vi "Wire Between Unbundle And Bundle For Message Converter With Oneof.vi"(8 "error in (no error)":errorcluster, 9 "Message Metadata":T1, 10 "VI Refnum":refnum<vi>, 11 "Library ref in":refnum<vi>) -> (0 "error IO":errorcluster, 2 "VI Refnum out":refnum<vi>, 3 "Library ref out":refnum<vi>)   [LabVIEW 2019, in "gRPC Template Creation Utility.lvlib"]
uses:
  gRPC Template Creation Utility.lvlib
  TypeDefs/Message Metadata (Scripting).ctl
  TypeDefs/Message Element Metadata (Scripting).ctl
  TypeDefs/Message Element Type.ctl
  <vilib>/Utility/miscctls.llb/LVPointTypeDef.ctl
  <vilib>/Utility/Data Type/NI_Data Type.lvlib
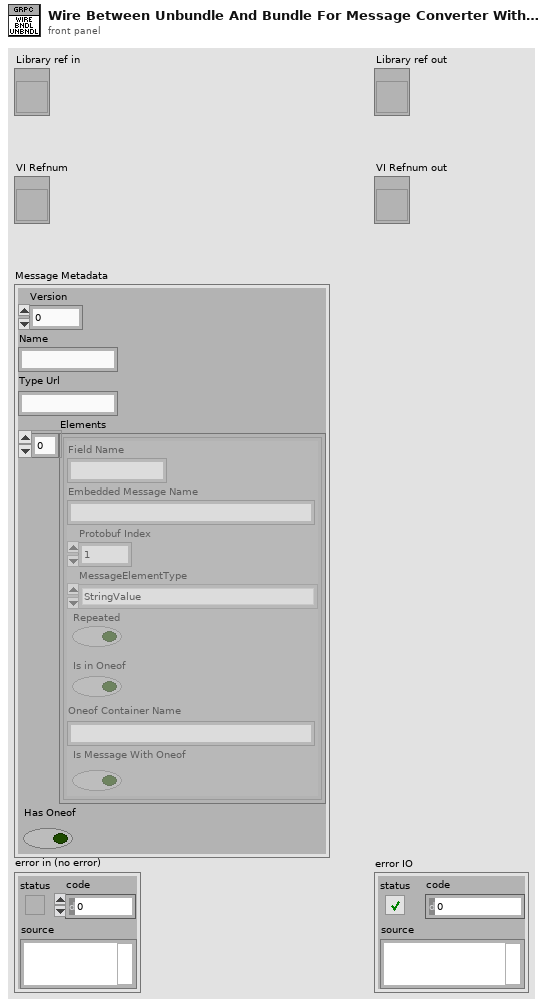
[diagram p1: front panel]
types:
  T1 = typedef "gRPC Template Creation Utility.lvlib/Message Metadata (Scripting).ctl" = cluster{"Version":i32, "Name":string, "Type Url":string, "Elements":T2[], "Has Oneof":bool}
  T2 = typedef "gRPC Template Creation Utility.lvlib/Message Element Metadata (Scripting).ctl" = cluster{"Field Name":string, "Embedded Message Name":string, "Protobuf Index":i32, "MessageElementType":T3, "Repeated":bool, "Is in Oneof":bool, "Oneof Container Name":string, "Is Message With Oneof":bool}
  T3 = typedef "gRPC Template Creation Utility.lvlib/Message Element Type.ctl" = enum32{"Int32Value", "FloatValue", "DoubleValue", "BoolValue", "StringValue", "MessageValue", "Int64Value", "UInt32Value", "UInt64Value", "EnumValue", "Bytes", "Fixed64", "Fixed32", "SFixed64", "SFixed32", "SInt64", "SInt32"}
  T4 = typedef "LVPointTypeDef.ctl" = cluster{"Horizontal":i16, "Vertical":i16}
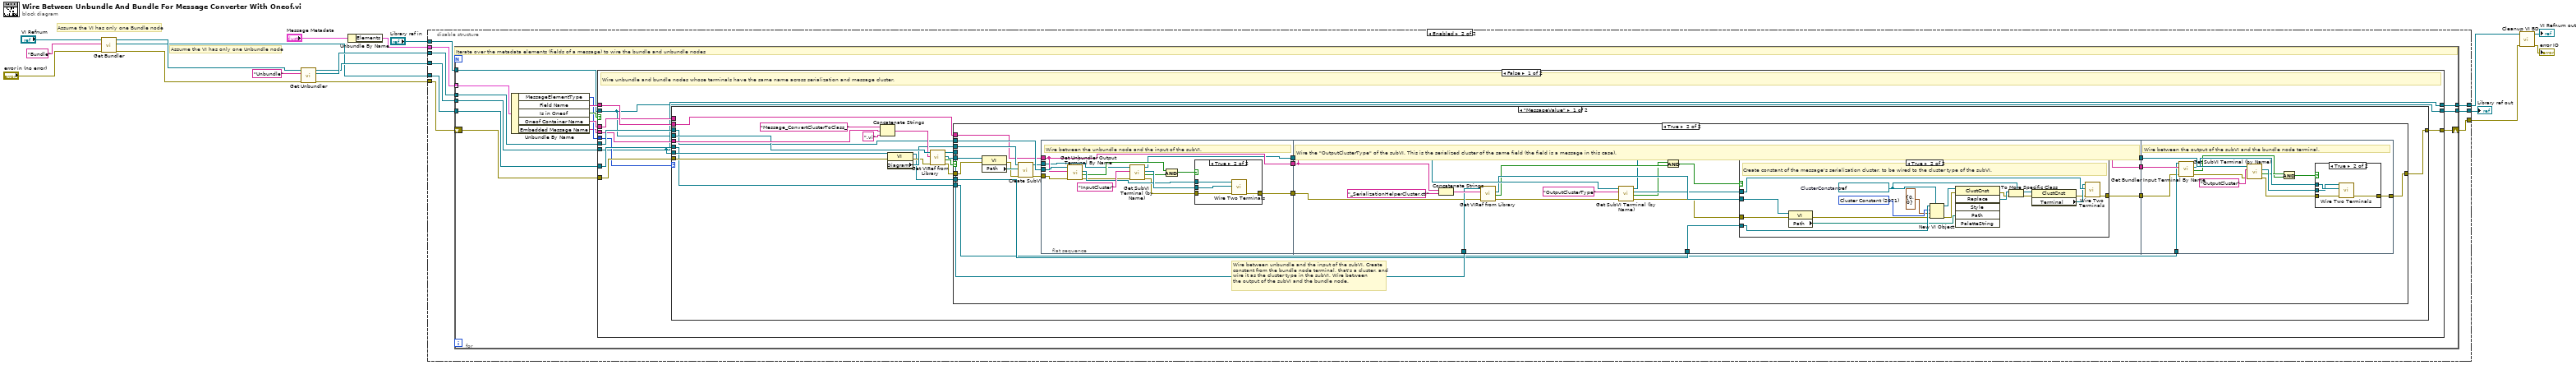
[diagram p0: block diagram]
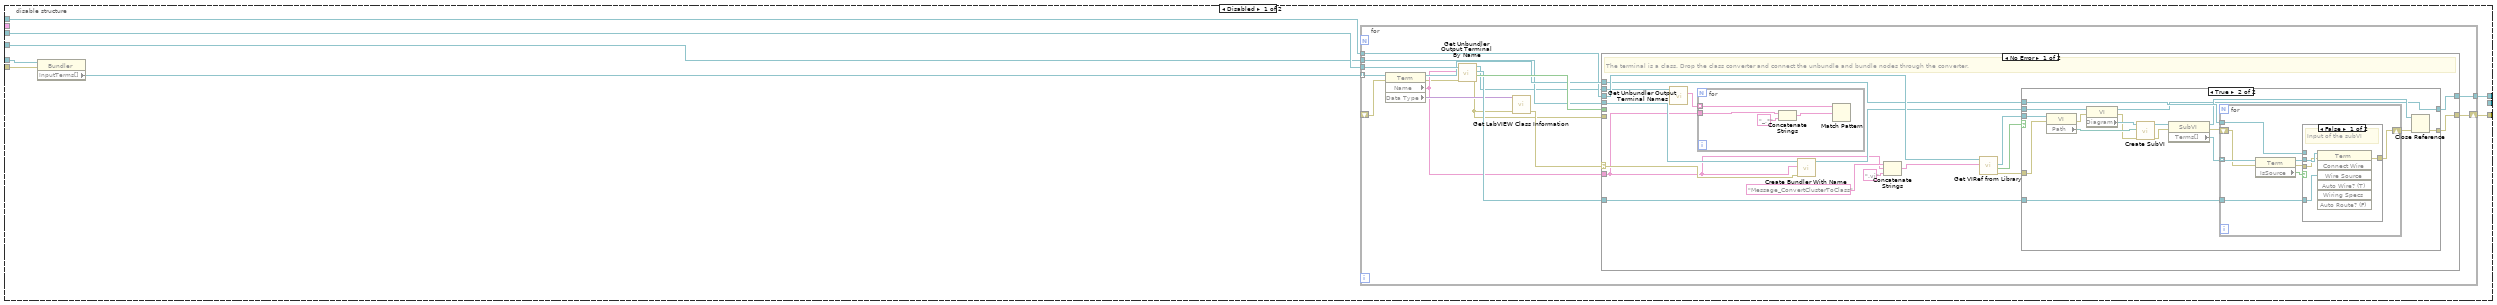
[diagram p2: hidden frame]
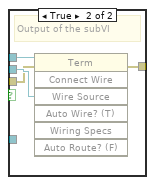
[diagram p4: hidden frame]
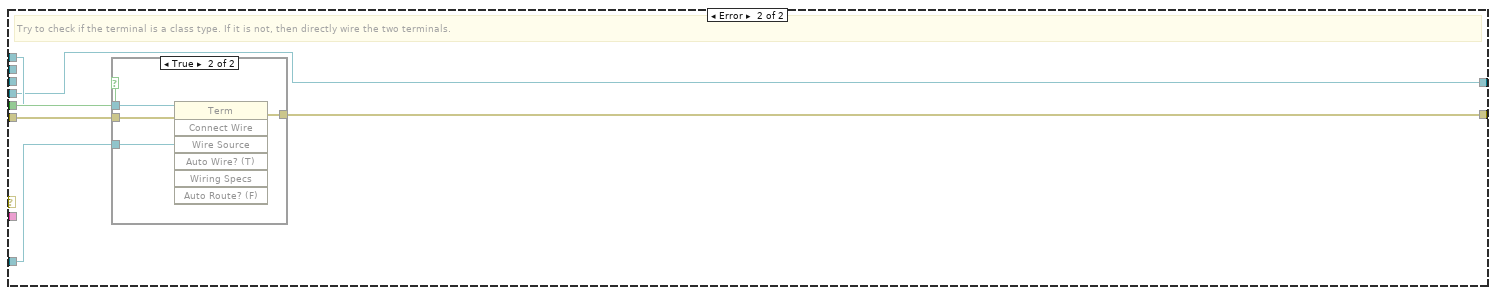
[diagram p5: hidden frame]
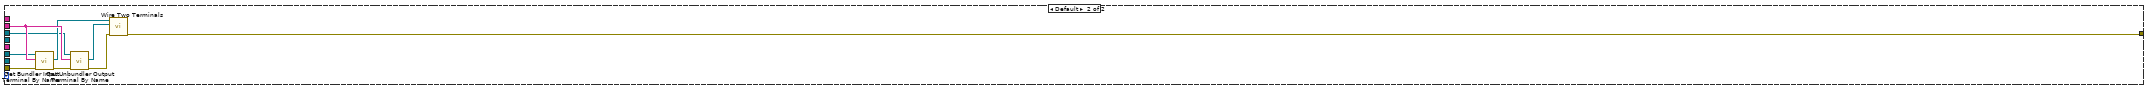
[diagram p11: hidden frame]
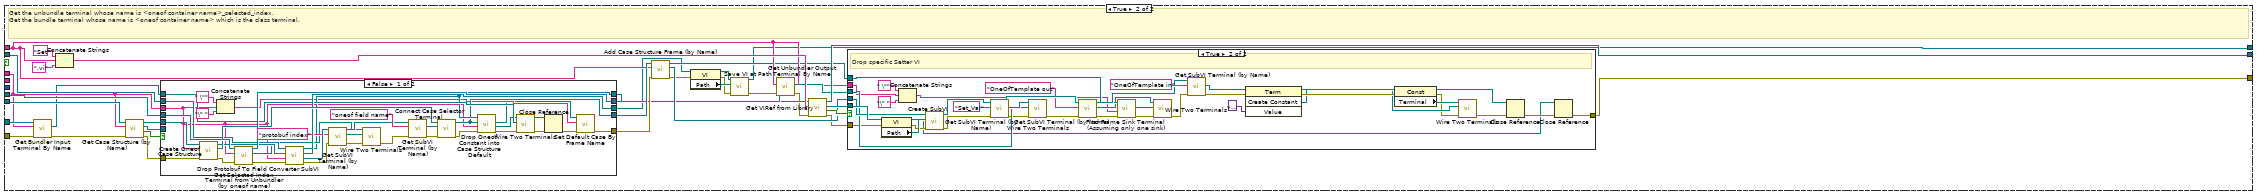
[diagram p12: hidden frame]
diagram:
  # "Assume the VI has only one Bundle node"
  # "Assume the VI has only one Unbundle node"
  n1 = call "Get Bundler.vi"("error in (no error)"="error in (no error)", "Label"="Bundle" ("Class Name"), "Owner VI in"="VI Refnum") -> ("error out"=w6:errorcluster, "Bundler ref out"=w3:refnum<vi>, "Owner VI out"=w7:refnum<vi>)  [unwired: 5 in, 1 out]
  n2 = call "Get Unbundler.vi"("error in (no error)"=w6, "Label"="Unbundle" ("Class Name"), "Owner VI in"=w7) -> ("error out"=w2:errorcluster, "Unbundler Refnum"=w9:refnum<vi>, "Owner VI out"=w8:refnum<vi>)  [unwired: 5 in, 1 out]
  n3 = Unbundle By Name("Message Metadata") -> ("Elements"=w4:T2[])
  n4 = disable-structure shown="Enabled" {
    disable-tunnel: "Library ref in" -> [w26 w114]
    disable-tunnel: [w25 w110] -> w16
    disable-tunnel: [w24 w112] -> w15
    disable-tunnel: w9 -> [w23 w116]
    disable-tunnel: w8 -> [w22 w115]
    disable-tunnel: [_ w113] -> w1
    disable-tunnel: w4 -> [_ w118]
    disable-tunnel: w3 -> [w21 w117]
    disable-tunnel: w2 -> [w20 w111]
    frame Disabled {
      n5 = property class="Bundler"(reference=w21, error in=w20) -> ("InputTerms[]"=w19:refnum<vi>[])  [unwired: 2 out]
      n6 = for {
        tunnel: w19 -> [w42] mode=indexing
        tunnel: w23 -> [w41]
        tunnel: w26 -> [w35]
        tunnel: w22 -> [w33]
        shift-right: [w31] -> w24
        shift-left: _ -> [w29]
        tunnel: [w28] -> w25
        n7 = property class="Term"(reference=w42, error in=w29) -> (reference out=w38:refnum<vi>, error out=w32:errorcluster, "Name"=w34:string, "Data Type"=w37:variant)
        n8 = call "Get Unbundler Output Terminal By Name.vi"("error in (no error)"=w32, "Terminal name"=w34, "Unbundler in"=w41) -> ("error out"=w30:errorcluster, "Found?"=w40:bool, "Terminal Refnum"=w39:refnum<vi>, "Unbundler out"=w27:refnum<vi>)  [unwired: 5 in]
        n9 = call <vilib>:"Get LabVIEW Class Information.vi"("error in (no error)"=w30, "variant"=w37) -> ("error out"=w36:errorcluster)  [unwired: 7 in, 2 out]
        n10 = case shown="No Error" w36 {
          selector: w36 -> [w47 _]
          tunnel: w40 -> [_ w104]
          tunnel: w39 -> [w53 w103]
          tunnel: w38 -> [w52 w102]
          tunnel: w35 -> [w59 _]
          tunnel: w34 -> [w43 _]
          tunnel: w33 -> [w48 w99]
          tunnel: [w50 w100] -> w31
          tunnel: w30 -> [_ w101]
          tunnel: [w49 w99] -> w28
          tunnel: w27 -> [w45 _]
          frame No Error {
            # "The terminal is a class. Drop the class converter and connect the unbundle and bundle nodes through the converter."
            n11 = call "Get Unbundler Output Terminal Names.vi"("Unbundler in"=w45) -> ("Terminal names"=w44:string[])  [unwired: 8 in, 2 out]
            n12 = for {
              tunnel: w44 -> [w63] mode=indexing
              tunnel: w43 -> [w60]
              n13 = Concatenate Strings(w60, "_.*" ("regular expression")) -> (w61:string)
              n14 = Match Pattern(string=w63, regular expression=w61) -> ()  [unwired: 1 in, 4 out]
            }
            n15 = call "Create Bundler With Name.vi"("error in (no error)"=w47, "Bundler Label"=w43, "VI in"=w48) -> ("VI out"=w46:refnum<vi>)  [unwired: 6 in, 2 out]
            n16 = Concatenate Strings("Message_ConvertClusterToClass" ("string"), w43, ".vi" ("string")) -> (w56:string)
            n17 = call "Get VIRef from Library.vi"("Item Name"=w56, "Library"=w59) -> ("error out"=w51:errorcluster, "Found ?"=w55:bool, "VIref out"=w54:refnum<vi>)  [unwired: 6 in, 1 out]
            n18 = case shown="True" w55 {
              tunnel: w54 -> [_ w82]
              tunnel: w46 -> [w64 w80]
              tunnel: w53 -> [_ w75]
              tunnel: w52 -> [_ w74]
              tunnel: w51 -> [w65 w71]
              tunnel: [w65 w67] -> w50
              tunnel: [w64 w66] -> w49
              frame False {
              }
              frame True {
                n19 = property class="VI"(reference=w82, error in=w71) -> (error out=w73:errorcluster, "Path"=w81:path)  [unwired: 1 out]
                n20 = property class="VI"(reference=w80, error in=w73) -> (reference out=w66:refnum<vi>, error out=w72:errorcluster, "Diagram"=w79:refnum<vi>)
                n21 = call "Create SubVI.vi"("error in (no error)"=w72, "Path"=w81, "Diagram in"=w79) -> ("error out"=w77:errorcluster, "subVI refnum"=w78:refnum<vi>)  [unwired: 7 in]
                n22 = property class="SubVI"(reference=w78, error in=w77) -> (reference out=w69:refnum<vi>, error out=w70:errorcluster, "Terms[]"=w76:refnum<vi>[])
                n23 = for {
                  tunnel: w76 -> [w90] mode=indexing
                  tunnel: w75 -> [w87]
                  tunnel: w74 -> [w86]
                  shift-right: [w83] -> w68
                  shift-left: w70 -> [w85]
                  n24 = property class="Term"(reference=w90, error in=w85) -> (reference out=w88:refnum<vi>, error out=w84:errorcluster, "IsSource"=w89:bool)
                  n25 = case shown="False" w89 {
                    tunnel: w88 -> [w94 w98]
                    tunnel: w87 -> [w93 _]
                    tunnel: w86 -> [_ w97]
                    tunnel: w84 -> [w92 w96]
                    tunnel: [w91 w95] -> w83
                    frame False {
                      # "Input of the subVI"
                      n26 = invoke class="Term" method="Connect Wire"(reference=w94, error in=w92, "Wire Source"=w93) -> (error out=w91:errorcluster)  [unwired: 4 in, 6 out]
                    }
                    frame True {
                      # "Output of the subVI"
                      n27 = invoke class="Term" method="Connect Wire"(reference=w97, error in=w96, "Wire Source"=w98) -> (error out=w95:errorcluster)  [unwired: 4 in, 6 out]
                    }
                  }
                }
                n28 = Close Reference(reference=w69, error in (no error)=w68) -> (error out=w67:errorcluster)
              }
            }
          }
          frame Error {
            # "Try to check if the terminal is a class type. If it is not, then directly wire the two terminals."
            n29 = case shown="True" w104 {
              tunnel: w103 -> [_ w108]
              tunnel: w102 -> [_ w109]
              tunnel: w101 -> [w105 w107]
              tunnel: [w105 w106] -> w100
              frame False {
              }
              frame True {
                n30 = invoke class="Term" method="Connect Wire"(reference=w109, error in=w107, "Wire Source"=w108) -> (error out=w106:errorcluster)  [unwired: 4 in, 6 out]
              }
            }
          }
        }
      }
    }
    frame Enabled {
      n31 = for {
        tunnel: w118 -> [w132] mode=indexing
        tunnel: w117 -> [w128]
        tunnel: w116 -> [w127]
        tunnel: w115 -> [w126]
        tunnel: w114 -> [w125]
        tunnel: [w124] -> w113
        shift-right: [w123] -> w112
        shift-left: w111 -> [w122]
        tunnel: [w121] -> w110
        # "Iterate over the metadata elements (fields of a message) to wire the bundle and unbundle nodes"
        n32 = Unbundle By Name(w132) -> ("MessageElementType"=w120:T3, "Field Name"=w129:string, "Is in Oneof"=w131:bool, "Oneof Container Name"=w130:string, "Embedded Message Name"=w119:string)
        n33 = case shown="False" w131 {
          tunnel: w130 -> [w136 w280]
          tunnel: w129 -> [w142 w272]
          tunnel: w122 -> [w141 w273]
          tunnel: [w140 w278] -> w123
          tunnel: w128 -> [w139 w298]
          tunnel: w127 -> [w138 w297]
          tunnel: w126 -> [w134 w296]
          tunnel: w125 -> [w133 w277]
          tunnel: [w133 w288] -> w124
          tunnel: [w134 w265] -> w121
          tunnel: w120 -> [w137 _]
          tunnel: w119 -> [w135 _]
          frame False {
            # "Wire unbundle and bundle nodes whose terminals have the same name across serialization and message cluster."
            n34 = case shown="\"MessageValue\"" w137 {
              tunnel: w142 -> [w147 w262]
              tunnel: w141 -> [w150 w260]
              tunnel: [w143 w257] -> w140
              tunnel: w139 -> [w144 w255]
              tunnel: w138 -> [w148 w254]
              tunnel: w136 -> [_ _]
              tunnel: w135 -> [w159 _]
              tunnel: w134 -> [w157 _]
              tunnel: w133 -> [w156 _]
              frame "MessageValue" {
                n35 = Concatenate Strings("Message_ConvertClusterToClass_", w159, ".vi" ("string")) -> (w155:string)
                n36 = property class="VI"(reference=w157, error in=w150) -> (reference out=w145:refnum<vi>, error out=w149:errorcluster, "Diagram"=w152:refnum<vi>)
                n37 = call "Get VIRef from Library.vi"("error in (no error)"=w149, "Item Name"=w155, "Library"=w156) -> ("error out"=w151:errorcluster, "Found ?"=w154:bool, "VIref out"=w153:refnum<vi>, "Library"=w146:refnum<vi>)  [unwired: 5 in]
                n38 = case shown="True" w154 {
                  tunnel: w153 -> [_ w180]
                  tunnel: w152 -> [_ w179]
                  tunnel: w151 -> [w161 w177]
                  tunnel: w148 -> [_ w175]
                  tunnel: w147 -> [_ w174]
                  tunnel: w146 -> [_ w172]
                  tunnel: w145 -> [_ w169]
                  tunnel: w144 -> [_ w167]
                  tunnel: [w161 w162] -> w143
                  frame False {
                  }
                  frame True {
                    # "Wire between unbundle and the input of the subVI. Create\nconstant from the bundle node terminal, that's a cluster, and\nwire it as the cluster type in the subVI. Wire between\nthe output of the subVI and the bundle node."
                    n39 = property class="VI"(reference=w180, error in=w177) -> (error out=w176:errorcluster, "Path"=w178:path)  [unwired: 1 out]
                    n40 = call "Create SubVI.vi"("error in (no error)"=w176, "Path"=w178, "Diagram in"=w179) -> ("error out"=w165:errorcluster, "subVI refnum"=w170:refnum<vi>)  [unwired: 7 in]
                    n41 = flat-sequence {
                      tunnel: w175 -> [w194]
                      tunnel: w174 -> [w187]
                      tunnel: [w187] -> w173
                      tunnel: [w186] -> w171
                      tunnel: w170 -> [w185]
                      tunnel: w165 -> [w184]
                      tunnel: [w181] -> w164
                      tunnel: w173 -> [w205]
                      tunnel: w172 -> [w214]
                      tunnel: w171 -> [w212]
                      tunnel: w169 -> [w209]
                      tunnel: [w205] -> w168
                      tunnel: [w204] -> w166
                      tunnel: w164 -> [w203]
                      tunnel: [w200] -> w163
                      tunnel: w168 -> [w248]
                      tunnel: w167 -> [w247]
                      tunnel: w166 -> [w246]
                      tunnel: w163 -> [w239]
                      tunnel: [w236] -> w162
                      frame #0 {
                        # "Wire between the unbundle node and the input of the subVI."
                        n42 = call "Get Unbundler Output Terminal By Name.vi"("error in (no error)"=w184, "Terminal name"=w187, "Unbundler in"=w194) -> ("error out"=w183:errorcluster, "Found?"=w189:bool, "Terminal Refnum"=w191:refnum<vi>)  [unwired: 5 in, 1 out]
                        n43 = call "Get SubVI Terminal (by Name).vi"("error in (no error)"=w183, "Terminal name"="InputCluster", "SubVI in"=w185) -> ("error out"=w182:errorcluster, "Found?"=w190:bool, "SubVI Term ref"=w192:refnum<vi>, "SubVI out"=w186:refnum<vi>)  [unwired: 5 in]
                        n44 = And(x=w189, y=w190) -> (x .and. y?=w188:bool)
                        n45 = case shown="True" w188 {
                          tunnel: w192 -> [_ w199]
                          tunnel: w191 -> [_ w198]
                          tunnel: w182 -> [w195 w197]
                          tunnel: [w195 w196] -> w181
                          frame False {
                          }
                          frame True {
                            n46 = call "Wire Two Terminals.vi"("error in (no error)"=w197, "Sink Terminal in"=w199, "Source Terminal"=w198) -> ("error out"=w196:errorcluster)  [unwired: 7 in, 1 out]
                          }
                        }
                      }
                      frame #1 {
                        # "Wire the \"OutputClusterType\" of the subVI. This is the serialized cluster of the same field (the field is a message in this case)."
                        n47 = Concatenate Strings(w205, "_SerializationHelperCluster.ctl" ("string")) -> (w215:string)
                        n48 = call "Get VIRef from Library.vi"("error in (no error)"=w203, "Item Name"=w215, "Library"=w214) -> ("error out"=w202:errorcluster, "Found ?"=w210:bool, "VIref out"=w211:refnum<vi>)  [unwired: 5 in, 1 out]
                        n49 = call "Get SubVI Terminal (by Name).vi"("error in (no error)"=w202, "Terminal name"="OutputClusterType", "SubVI in"=w212) -> ("error out"=w201:errorcluster, "Found?"=w206:bool, "SubVI Term ref"=w208:refnum<vi>, "SubVI out"=w204:refnum<vi>)  [unwired: 5 in]
                        n50 = And(x=w206, y=w210) -> (x .and. y?=w207:bool)
                        n51 = case shown="True" w207 {
                          tunnel: w211 -> [_ w235]
                          tunnel: w209 -> [_ w234]
                          tunnel: w208 -> [_ w229]
                          tunnel: w201 -> [w217 w224]
                          tunnel: [w217 w218] -> w200
                          frame False {
                          }
                          frame True {
                            w227 = refnum<vi> refnum  # ClusterConstant
                            w233 = 2071 items=[".NET Container"=2125, ".NET Refnum"=3441, "2D Picture"=3508, "3D Picture"=23776, "Absolute Value"=1054, "Accept TLS"=1732, "Access Rights"=1412, "ActiveX Container"=2072, "Add"=1050, "Add (with error terminals)"=3915, "Add Array Elements"=1903, "Add Entropy"=1738, "Add Private Key To TLS Configuration"=1735, "Add Trusted Certificate To TLS Configuration"=1736, "Agitator"=3831, "AllSpoll"=1960, "Always Copy"=2400, "And"=1061, "And Array Elements"=1911, "Append True/False String"=1511, "Application Refnum"=3412, "Array (block diagram constant)"=2070, "Array (classic)"=3300, "Array (modern)"=21608, "Array Interface Control"=23777, "Array Max & Min"=1907, "Array of Strings to Path"=1422, "Array Size"=1809, "Array Subset"=2044, "Array To Cluster"=1168, "Array To Spreadsheet String"=1540, "ArrayMemInfo"=2412, "Assert Structural Type Match"=2416, "Assert Structural Type Mismatch"=2464, "Atmospheric Tank (classic)"=3070, "Atmospheric Tank (modern)"=21751, "Automation Close"=8001, "Automation Open"=8000, "Automation Refnum"=3410, "Avogadro Constant (1/mol)"=23520, "Base 10 Logarithm Of e"=23512, "Bin #1"=3073, "Bin #2"=21755, "Bitpack to Array"=3135, "Bluetooth Close Connection"=9148, "Bluetooth Create Listener"=9151, "Bluetooth Discover"=9152, "Bluetooth Network Connection Refnum"=3468, "Bluetooth Open Connection"=9153, "Bluetooth Read"=9149, "Bluetooth Wait On Listener"=9147, "Bluetooth Write"=9150, "Boolean Array To Number"=1815, "Boolean To (0,1)"=1167, "Build Array"=2041, "Build Cluster Array"=2047, "Build Map"=2463, "Build Matrix"=8500, "Build Path"=1419, "Build Set"=2462, "Build Waveform"=2066, "Bundle"=2049, "Bundle By Name"=2057, "Byte Array To String"=1609, "Byte Stream File Refnum"=3408, "Call By Reference"=3901, "Call Chain"=1999, "Call Library Function Node"=2062, "Call Parent Method"=2354, "CAN Channel (block diagram constant)"=2124, "CAN Channel (classic)"=3340, "CAN Channel (modern)"=21817, "CAN Channel (system)"=21966, "CAN Interface (block diagram constant)"=2123, "CAN Interface (classic)"=3339, "CAN Interface (modern)"=21815, "CAN Interface (system)"=21964, "CAN Task (block diagram constant)"=3471, "CAN Task (classic)"=3470, "CAN Task (modern)"=21789, "CAN Task (system)"=21963, "Cancel Button (modern)"=21739, "Cancel Button (system)"=3131, "Cancel Notification"=9107, "Carriage Return Constant"=23500, "Case Structure"=2001, "Cast Unit Bases"=1079, "Check Valve"=3833, "Checkbox (classic)"=3117, "CheckBox (modern)"=21924, "Checkbox (system)"=3132, "Class Specifier Constant"=2094, "Classic Color Box"=3013, "Classic Color Ramp"=3022, "Classic Horizontal Slide Switch"=3114, "Classic Vertical Slide"=3004, "Clear Fixed-Point Overflow Status"=5562, "Close File"=8052, "Close File (deprecated)"=1405, "Close Python Session"=24207, "Close Reference"=8011, "Close Variable Connection"=23783, "Closure Structure"=2372, "Cluster (classic)"=3400, "Cluster (modern)"=21607, "Cluster Constant"=2071, "Cluster To Array"=1169, "Code Interface Node"=2050, "Coerce To Type"=2402, "Collection Size"=2450, "Color Box Constant"=2120, "Color Box Thin Border"=2905, "Colored Rectangle (broken?)"=3625, "Combo Box (classic)"=3304, "Combo Box (modern)"=21604, "Combo Box (system)"=21917, "Combo Box Constant"=2088, "Complex Conjugate"=1048, "Complex To Polar"=1045, "Complex To Re/Im"=1044, "Compound Arithmetic"=2200, "Compressor"=3832, "Concatenate Strings"=2040, "Conditional Disable Structure"=2064, "Constructor Node"=3904, "Control & Simulation Loop"=2099, "Control Help Window"=1353, "Control Online Help"=1355, "Control Refnum"=3419, "Convert Unit"=2059, "Conveyer"=3827, "Copy"=8053, "Copy (deprecated)"=1416, "Cosecant"=1204, "Cosine"=1201, "Cotangent"=1205, "CPU Information"=24130, "Create Folder"=8055, "Create Network Stream Endpoint"=23793, "Create Network Stream Reader Endpoint"=23811, "Create Network Stream Writer Endpoint"=23810, "Create Stream"=23796, "Create Unique Network Stream Endpoint"=23795, "Create Unique Network Stream Reader Endpoint"=23807, "Create Unique Network Stream Writer Endpoint"=23806, "Create User Event"=2073, "Current Processor ID"=24131, "Current VI's Menubar"=9000, "Current VI's Path"=1426, "DAQmx Analog Trigger Source (block diagram constant)"=2119, "DAQmx Analog Trigger Source (classic)"=3336, "DAQmx Analog Trigger Source (modern)"=21774, "DAQmx Analog Trigger Source (system)"=21951, "DAQmx Device Name (block diagram constant)"=2093, "DAQmx Device Name (classic)"=3318, "DAQmx Device Name (modern)"=21773, "DAQmx Device Name (system)"=21950, "DAQmx Global Channel (block diagram constant)"=3430, "DAQmx Global Channel (classic)"=3443, "DAQmx Global Channel (modern)"=21770, "DAQmx Global Channel (system)"=21957, "DAQmx Physical Channel (block diagram constant)"=2118, "DAQmx Physical Channel (classic)"=3335, "DAQmx Physical Channel (modern)"=21777, "DAQmx Physical Channel (system)"=21954, "DAQmx Scale Name (block diagram constant)"=2116, "DAQmx Scale Name (classic)"=3317, "DAQmx Scale Name (modern)"=21775, "DAQmx Scale Name (system)"=21952, "DAQmx Switch (block diagram constant)"=2121, "DAQmx Switch (classic)"=3337, "DAQmx Switch (modern)"=21776, "DAQmx Switch (system)"=21953, "DAQmx Task Name (block diagram constant)"=3434, "DAQmx Task Name (classic)"=3442, "DAQmx Task Name (modern)"=21778, "DAQmx Task Name (system)"=21959, "DAQmx Terminal (block diagram constant)"=2117, "DAQmx Terminal (classic)"=3319, "DAQmx Terminal (modern)"=21781, "DAQmx Terminal (system)"=21955, "Data Cache Size"=24132, "Data Log File Refnum"=3402, "Data Value Reference"=3476, "Data Value Reference Constant"=24134, "DataSocket Close"=1085, "DataSocket Open"=1084, "DataSocket Read"=1086, "DataSocket Refnum"=3417, "DataSocket Write"=1087, "Date/Time To Seconds"=1308, "Decimal Digit?"=1119, "Decimal String To Number"=1184, "Decimate 1D Array"=2046, "DecomposeLockDataValRef"=2406, "DecomposeVariant"=2404, "Decrement"=1058, "Default Directory"=1427, "Delete"=8056, "Delete (deprecated)"=1417, "Delete Data Value Reference"=2409, "Delete From Array"=3912, "Delete Menu Items"=9004, "Delete Variant Attribute"=8206, "Delete Waveform Attribute"=8209, "Deny Access"=8057, "Dequeue Element"=9113, "Destroy Stream Endpoint"=23794, "Destroy User Event"=2075, "DevClear"=1961, "DevClearList"=1962, "Device Control/Status"=1433, "Device Refnum"=3405, "Diagram Disable Structure"=2054, "Dial (classic)"=3050, "Dial (modern)"=21732, "Digital Data (classic)"=3210, "Digital Data (modern)"=21216, "Digital Waveform Graph (classic)"=3511, "Digital Waveform Graph (modern)"=21718, "Direct Variable Read"=23785, "Direct Variable Write"=23788, "Divide"=1053, "Divide (with error terminals)"=3918, "Dlg Horiz Scrollbar"=21905, "Dlg Mac Group Box"=32514, "Dlg Numeric #1"=2100, "Dlg Numeric #2"=3006, "Dlg String"=2110, "Dlg Vert Scrollbar"=21906, "Down Arrow"=3824, "Down Bow Valve (flat)"=3707, "Down Bow Valve (outline)"=3807, "Down Bow Valve (shaded)"=21767, "Down Rect Valve (flat)"=3706, "Down Rect Valve (outline)"=3806, "Down Rect Valve (shaded)"=21766, "Down Tee (flat)"=3818, "Down Tee (shaded)"=3718, "Dynamic FPGA Interface Cast"=5690, "Eased Corner Rectangle"=32513, "Element of Set?"=2454, "Elementary Charge (C)"=23517, "Empty Array?"=23063, "Empty Collection?"=2451, "Empty Path Constant"=23523, "Empty String Constant"=23503, "Empty String/Path?"=1112, "Enable Menu Tracking"=9002, "EnableLocal"=1963, "EnableRemote"=1964, "End of Line Constant"=23525, "Enqueue Element"=9111, "Enqueue Element At Opposite End"=9129, "Enum (classic)"=3023, "Enum (modern)"=21605, "Enum (system)"=3062, "Enum Constant"=2090, "EOF"=1410, "Equal To 0?"=1113, "Equal?"=1102, "Error Ring Constant"=2039, "Event Callback Refnum"=3435, "Event Data Node"=2102, "Event Structure"=2052, "Exchanger"=3828, "Exclusive Or"=1063, "Exponential"=1211, "Exponential (Arg) -1"=1222, "Expression Node"=2201, "False Constant"=2006, "Feedback Node"=2353, "FieldPoint IO Point (block diagram constant)"=3440, "FieldPoint IO Point (classic)"=3439, "FieldPoint IO Point (modern)"=21784, "FIFO Refnum"=3474, "File Dialog"=8058, "File Dialog (deprecated)"=8081, "File Path Control (classic)"=3203, "File Path Control (modern)"=21730, "File Path Control (system)"=21922, "File Path Indicator (classic)"=3204, "File Path Indicator (modern)"=21731, "File/Directory Info"=8082, "File/Directory Info (deprecated)"=1413, "FindLstn"=1965, "FindRQS"=1966, "First Call?"=1083, "Fixed-Point Overflow?"=5565, "Fixed-Point to Integer Cast"=5566, "Flat Box"=3602, "Flat Circle"=3605, "Flat Down Triangle"=3623, "Flat Frame"=3608, "Flat Left Triangle"=3620, "Flat Right Triangle"=3621, "Flat Round Button"=3102, "Flat Rounded Box"=3611, "Flat Sequence Structure"=2069, "Flat Square Button"=3103, "Flat Up Triangle"=3622, "Flatten To JSON"=24201, "Flatten To String"=1164, "Flatten To XML"=8400, "Flattened String To Variant"=8202, "Floating Point Equal?"=23064, "Flush Event Queue"=2135, "Flush File"=8059, "Flush File (deprecated)"=1406, "Flush Queue"=9114, "Flush Stream"=23808, "For Loop"=2002, "Fork"=2194, "Format Date/Time String"=8100, "Format Into File"=2083, "Format Into String"=2081, "Format Value"=1512, "Formula Node"=2004, "FPGA Refnum to Session"=2322, "Fract/Exp String To Number"=1187, "Framed Color Box (classic)"=3008, "Framed Color Box (modern)"=21019, "Free Label"=2321, "Furnace"=3829, "Gauge (classic)"=3040, "Gauge (modern)"=21009, "Gauge for Simon"=32600, "Generate Front Panel Activity"=1329, "Generate Occurrence"=1700, "Generate User Event"=2074, "Generate User-Defined Trace Event"=2250, "Get Control Values by Index"=24204, "Get Datalog Position"=8061, "Get Date/Time In Seconds"=1303, "Get Date/Time String"=1600, "Get Drag Drop Data"=9154, "Get File Position"=8062, "Get File Size"=8063, "Get Fixed-Point Components"=11163, "Get Help Window Status"=1354, "Get Matrix Diagonal"=8501, "Get Matrix Elements"=8502, "Get Menu Item Info"=9005, "Get Menu Selection"=9001, "Get Menu Short Cut Info"=9007, "Get Notifier Status"=9103, "Get Number of Records"=8064, "Get Permissions"=8065, "Get Queue Status"=9110, "Get Submatrix"=8503, "Get Type and Creator"=8066, "Get Variant Attribute"=8205, "Get Volume Info"=8067, "Get Waveform Attribute"=8208, "Get Waveform Components"=2067, "Global Variable"=2060, "GPIB Clear"=1954, "GPIB Initialization"=1957, "GPIB Misc"=1956, "GPIB Read"=1951, "GPIB Serial Poll"=1955, "GPIB Status"=1959, "GPIB Trigger"=1953, "GPIB Wait"=1958, "GPIB Write"=1950, "Gravitational Constant (N m2/kg2)"=23519, "Greater Or Equal To 0?"=1114, "Greater Or Equal?"=1103, "Greater Than 0?"=1117, "Greater?"=1110, "Handle Peek"=1604, "Handle Poke"=1605, "Hex Digit?"=1123, "Hexadecimal String To Number"=1185, "Hopper #1"=21754, "Hopper #2"=3072, "Horiz Line"=3821, "Horiz Pipe (flat)"=3810, "Horiz Pipe (shaded)"=3710, "Horizontal Button Box"=3636, "Horizontal Fill Slide (classic)"=3012, "Horizontal Fill Slide (modern)"=21100, "Horizontal Gradient Oval"=32502, "Horizontal Gradient Rectangle"=32504, "Horizontal Gradient Rounded Rectangle"=32507, "Horizontal Graduated Bar"=21106, "Horizontal Pointer Slide (classic)"=3011, "Horizontal Pointer Slide (modern)"=21101, "Horizontal Pointer Slide (system)"=21902, "Horizontal Progress Bar (modern)"=21102, "Horizontal Progress Bar (system)"=21910, "Horizontal Scrollbar"=21110, "Horizontal Slide (classic)"=3010, "Horizontal Slide (system)"=21904, "Horizontal Smooth Box"=3633, "Horizontal Splitter Bar"=21861, "Horizontal Splitter Bar (Classic)"=21863, "Horizontal Splitter Bar (NXG Style)"=21867, "Horizontal Splitter Bar (System)"=21865, "Horizontal Switch"=3108, "Horizontal Tank"=3071, "Horizontal Toggle Switch (classic)"=3110, "Horizontal Toggle Switch (modern)"=21700, "Hyperbolic Cosecant"=23053, "Hyperbolic Cosine"=1215, "Hyperbolic Cotangent"=23055, "Hyperbolic Secant"=23054, "Hyperbolic Sine"=1214, "Hyperbolic Tangent"=1216, "IMAQ Session"=3415, "Implies"=1080, "In Place Element Structure"=2360, "In Range and Coerce"=1127, "Include Fixed-Point Overflow Status"=5564, "Increment"=1057, "Index & Bundle Cluster Array"=2056, "Index Array"=2042, "Index String Array"=1531, "Initialize Array"=2053, "Inline C Node"=2104, "Insert Into Array"=3911, "Insert Into Map"=2456, "Insert Into Set"=2452, "Insert Menu Items"=9003, "Integer to Fixed-Point Cast"=5567, "Intensity Chart (classic)"=3509, "Intensity Chart (modern)"=21719, "Intensity Graph (classic)"=3510, "Intensity Graph (modern)"=21720, "Interleave 1D Arrays"=2045, "Interpolate 1D Array"=1905, "Inverse Cosecant"=23050, "Inverse Cosine"=1207, "Inverse Cotangent"=23052, "Inverse Hyperbolic Cosecant"=23056, "Inverse Hyperbolic Cosine"=1218, "Inverse Hyperbolic Cotangent"=23058, "Inverse Hyperbolic Secant"=23057, "Inverse Hyperbolic Sine"=1217, "Inverse Hyperbolic Tangent"=1219, "Inverse Secant"=23051, "Inverse Sine"=1206, "Inverse Tangent"=1208, "Inverse Tangent (2 Input)"=1228, "Invoke Node"=3900, "IP To String"=1710, "IrDA Close Connection"=9144, "IrDA Create Listener"=9140, "IrDA Discover"=9141, "IrDA Network Connection Refnum"=3450, "IrDA Open Connection"=9142, "IrDA Read"=9145, "IrDA Wait On Listener"=9143, "IrDA Write"=9146, "IVI Delete Session"=8103, "IVI Logical Name (block diagram constant)"=3420, "IVI Logical Name (classic)"=3414, "IVI Logical Name (modern)"=21736, "IVI New Session"=8102, "Join"=2195, "Join Numbers"=1171, "Junction"=2197, "Knob (classic)"=3005, "Knob (modern)"=21000, "Label (modern)"=21960, "Label (system)"=21961, "Labeled Oblong Button"=3125, "Labeled Rectangular Button"=3124, "Labeled Round Button"=3122, "Labeled Square Button"=3123, "LabVIEW Object"=3457, "Leak Variant Value Reference"=2410, "LED Button"=3116, "Left Arrow"=3826, "Left Bow Valve (flat)"=3701, "Left Bow Valve (outline)"=3801, "Left Bow Valve (shaded)"=21761, "Left Down Elbow (flat)"=3811, "Left Down Elbow (shaded)"=3711, "Left Pump (flat)"=3813, "Left Pump (shaded)"=3713, "Left Rect Valve (flat)"=3700, "Left Rect Valve (outline)"=3800, "Left Rect Valve (shaded)"=21760, "Left Tee (flat)"=3809, "Left Tee (shaded)"=3709, "Left Up Elbow (flat)"=3808, "Left Up Elbow (shaded)"=3708, "Less Or Equal To 0?"=1115, "Less Or Equal?"=1104, "Less Than 0?"=1118, "Less?"=1111, "Lexical Class"=1126, "Line (chiseled, system)"=3632, "Line (chiseled, thick)"=3630, "Line (chiseled, thin)"=3627, "Line (thick)"=3629, "Line (thin)"=3626, "Line Feed Constant"=23501, "Line with Arrow (thick)"=3631, "Line with Arrow (thin)"=3628, "List Directory"=1418, "List Folder"=8083, "Listbox (classic)"=21806, "Listbox (modern)"=21792, "Listbox (system)"=21805, "Listbox Symbol Ring Constant"=2038, "Load Certificates Into Memory"=1734, "Load Private Key Into Memory"=1733, "Local Variable"=2061, "Lock Range"=1411, "Logarithm Base 10"=1210, "Logarithm Base 2"=1225, "Logarithm Base X"=1224, "Logical Shift"=1081, "Look In Map"=2458, "Lookup Channel Probe"=9155, "Lossy Enqueue Element"=9130, "Lowered Box (thick)"=3635, "Lowered Rounded Box"=3638, "Machine Epsilon"=23528, "Make TLS Configuration Immutable"=1737, "MakeAddr"=1967, "Mantissa & Exponent"=1150, "Map"=3488, "Map Constant"=2461, "Match First String"=1532, "Match Pattern"=1535, "Match True/False String"=1533, "MathScript Call By Reference"=3906, "MathScript Node"=2357, "MATLAB script"=9020, "Matrix Size"=8507, "Max & Min"=1108, "Menu Refnum"=3413, "Menu Ring (classic)"=3018, "Menu Ring (modern)"=21600, "Menu-Popup Ring"=3017, "Merge Errors"=2147, "Merge Signals"=2350, "Meter (classic)"=3030, "Meter (modern)"=21008, "Mixed Checkbox (system)"=21333, "Mixed Signal Graph"=21721, "Molar Gas Constant (J/(mol K))"=23522, "Motion Resource (block diagram constant)"=3449, "Motion Resource (classic)"=3448, "Motion Resource (modern)"=21787, "Motor (flat)"=3820, "Motor (shaded)"=3720, "Move"=8068, "Move (deprecated)"=1415, "Multi-Segment Pipe"=23780, "Multicolumn Listbox (classic)"=21799, "Multicolumn Listbox (modern)"=21791, "Multicolumn Listbox (system)"=21798, "Multiply"=1052, "Multiply (with error terminals)"=3917, "Multiply Array Elements"=1904, "Multirate Structure"=2199, "Natural Logarithm"=1209, "Natural Logarithm (Arg +1)"=1221, "Natural Logarithm Base"=23510, "Natural Logarithm Of 10"=23513, "Natural Logarithm Of 2"=23514, "Natural Logarithm Of Pi"=23508, "Negate"=1069, "Negative Infinity"=23509, "New Data Value Reference"=2408, "New Directory"=1402, "New File"=1404, "New TLS Configuration"=1730, "New VI"=8014, "New VI Object"=8015, "Not"=1064, "Not A Number/Path/Refnum?"=1128, "Not A Path Constant"=23524, "Not a Refnum Constant"=23526, "Not a Shared Variable"=23527, "Not And"=1071, "Not Equal To 0?"=1116, "Not Equal?"=1105, "Not Exclusive Or"=1073, "Not Or"=1072, "Notifier Refnum"=3423, "Number of Cache Levels"=24133, "Number To Boolean Array"=1814, "Number To Decimal String"=1180, "Number To Engineering String"=1183, "Number To Exponential String"=1505, "Number To Fractional String"=1506, "Number To Hexadecimal String"=1181, "Number To Octal String"=1182, "Numeric Constant"=2005, "Numeric Control (classic)"=3000, "Numeric Control (modern)"=21003, "Numeric Control (system)"=21919, "Numeric Indicator (classic)"=3001, "Numeric Indicator (modern)"=21004, "Obtain Notifier"=9101, "Obtain Queue"=9108, "Occurrence Refnum"=3406, "Octal Digit?"=1129, "Octal String To Number"=1186, "OK Button (modern)"=21738, "OK Button (system)"=3130, "Old VISA Open"=1921, "OLE Variant"=3150, "One Button Dialog"=1340, "Open and Verify Variable Connection"=23790, "Open Application Reference"=8012, "Open Device"=1430, "Open Dynamic Bitfile Reference"=5691, "Open File"=1403, "Open Python Session"=24206, "Open Tank (flat classic)"=21752, "Open Tank (shaded classic)"=3074, "Open Variable Connection"=23779, "Open Variable Connection in Background"=23791, "Open VI Object Reference"=8013, "Open VI Reference"=8010, "Open/Create/Replace Datalog"=8054, "Open/Create/Replace File"=8050, "Or"=1062, "Or Array Elements"=1910, "Oval with Shadow"=32509, "Package Matrix"=23001, "PassControl"=1968, "Path Constant"=2009, "Path to Array of Strings"=1423, "Path To String"=1077, "Path Type"=1421, "Pi"=23504, "Pi Divided By 2"=23506, "Pi Multiplied By 2"=23505, "Pick Line"=1510, "Pict Ring (classic)"=3015, "Pict Ring (modern)"=21602, "Pict Ring (system)"=21925, "PixMap"=3505, "PixMap (warning: dangerous)"=3507, "Planck's Constant (J/Hz)"=23516, "Platform Flat Square Button"=3134, "Plug-In Control"=21820, "Polar To Complex"=1047, "Polar To Re/Im"=23061, "Positive Infinity"=23515, "Power Of 10"=1212, "Power Of 2"=1223, "Power Of X"=1213, "PPoll"=1969, "PPollConfig"=1970, "PPollUnconfig"=1971, "Preallocated Read from Binary File"=24135, "Preserve Run-Time Class"=8018, "Pressure Tank (flat)"=3075, "Pressure Tank (shaded)"=21753, "Preview Queue Element"=9112, "Printable?"=1124, "Property Node"=1920, "Pulldown Menu Ring"=3061, "Push Button"=21001, "Python Node"=24205, "Python Session Refnum"=3486, "Queue Refnum"=3424, "Quit LabVIEW"=1352, "Quotient & Remainder"=1056, "Race Structure"=2371, "Radio Button (system)"=3133, "Radio Buttons (classic)"=22003, "Radio Buttons (modern)"=22001, "Radio Buttons (system)"=22002, "Raised Box (classic)"=3600, "Raised Box (modern)"=3637, "Raised Circle"=3603, "Raised Down Triangle"=3615, "Raised Frame"=3606, "Raised Left Triangle"=3612, "Raised Right Triangle"=3613, "Raised Rounded Box"=3609, "Raised Up Triangle"=3614, "Random Number (0-1)"=1070, "RcvRespMsg"=1972, "Re-accept TLS"=1739, "Re/Im To Complex"=1046, "Re/Im To Polar"=23060, "Read Datalog"=8069, "Read Device"=1432, "Read File"=1407, "Read from Binary File"=8051, "Read from Text File"=8070, "Read Map Max & Min Keys"=2459, "Read Multiple Elements from Stream"=23803, "Read Set Max & Min"=2455, "Read Single Element from Stream"=23797, "Read Variable"=23781, "Read Variable with Timeout"=23786, "ReadStatus"=1973, "Receive"=1974, "ReceiveSetup"=1975, "Recessed Box"=3601, "Recessed Circle"=3604, "Recessed Down Triangle"=3619, "Recessed Frame (modern)"=3607, "Recessed Frame (system)"=3624, "Recessed Left Triangle"=3616, "Recessed Menu Ring"=3019, "Recessed Right Triangle"=3617, "Recessed Rounded Box"=3610, "Recessed Up Triangle"=3618, "Reciprocal"=1059, "Reciprocal Of e"=23511, "Reciprocal Of Pi"=23507, "RecomposeArray"=2403, "RecomposeUnlockDataValRef (warning: dangerous)"=2407, "RecomposeVariant (warning: dangerous)"=2405, "Rectangular Stop Button"=3128, "Refnum to Path"=1424, "Refnum to Session"=2306, "Region"=2196, "Register Event Callback"=2078, "Register For Events"=2065, "Register Session"=2319, "Release Notifier"=9102, "Release Queue"=9109, "Remove Fixed-Point Overflow Status"=5563, "Remove From Map"=2457, "Remove From Set"=2453, "Replace Array Subset"=3910, "Replace Substring"=3913, "Request Deallocation"=1610, "ResetSys"=1976, "Reshape Array"=2055, "Resize Matrix"=8508, "Resource Index"=1088, "Reverse 1D Array"=1900, "Reverse String"=1537, "Right Arrow"=3825, "Right Bow Valve (flat)"=3705, "Right Bow Valve (outline)"=3805, "Right Bow Valve (shaded)"=21765, "Right Down Elbow (flat)"=3817, "Right Down Elbow (shaded)"=3717, "Right Pump (flat)"=3819, "Right Pump (shaded)"=3719, "Right Rect Valve (flat)"=3704, "Right Rect Valve (outline)"=3804, "Right Rect Valve (shaded)"=21764, "Right Tee (flat)"=3815, "Right Tee (shaded)"=3715, "Right Up Elbow (flat)"=3814, "Right Up Elbow (shaded)"=3714, "Rocker"=21002, "Rotary Feeder"=3830, "Rotate"=1082, "Rotate 1D Array"=1906, "Rotate Left With Carry"=1606, "Rotate Right With Carry"=1607, "Rotate String"=1536, "Round Button"=3100, "Round LED (classic)"=3120, "Round LED (modern)"=21012, "Round Light"=3104, "Round Push Button"=3118, "Round Push Button (profile)"=3112, "Round Radio Button"=3106, "Round Stop Button"=3127, "Round To Nearest"=1055, "Round Toward +Infinity"=1076, "Round Toward -Infinity"=1075, "Rounded Rectangle with Shadow"=32508, "RT FIFO Create"=24000, "RT FIFO Delete"=24003, "RT FIFO Read"=24001, "RT FIFO Write"=24002, "Rydberg Constant (1/m)"=23521, "Scale By Power Of 2"=1074, "Scan From File"=2082, "Scan From String"=2080, "Scan String For Tokens"=8101, "Scan Value"=1534, "Scanned Variable Read"=23784, "Scanned Variable Write"=23787, "Search 1D Array"=1901, "Search and Replace String"=3914, "Search Variable Container"=23802, "Search/Split String"=1538, "Secant"=1203, "Seconds To Date/Time"=1309, "Seek"=1409, "Select"=1516, "Send"=1977, "Send Notification"=9104, "SendCmds"=1978, "SendDataBytes"=1979, "SendIFC"=1980, "SendList"=1981, "SendLLO"=1982, "SendSetup"=1983, "Session to Refnum"=2307, "Set"=3487, "Set Constant"=2460, "Set Control Values by Index"=24203, "Set Datalog Position"=8072, "Set File Position"=8073, "Set File Size"=8074, "Set Matrix Diagonal"=8504, "Set Matrix Elements"=8505, "Set Menu Item Info"=9006, "Set Number of Records"=8075, "Set Occurrence"=1702, "Set Permissions"=8076, "Set Submatrix"=8506, "Set Type and Creator"=8077, "Set Variant Attribute"=8204, "Set Waveform Attribute"=8207, "SetRWLS"=1984, "SetTimeOut"=1985, "Shared Variable"=23778, "Shared Variable Constant"=3473, "Shared Variable Control (classic)"=3472, "Shared Variable Control (modern)"=21814, "Shared Variable to String"=1831, "Sign"=1049, "Simple Horizontal Slide"=3003, "Simple Numeric"=2900, "Simple String"=2115, "Simple Vertical Slide"=3002, "Sinc"=1227, "Sine"=1200, "Sine & Cosine"=1220, "Size Handle"=1603, "Slide Switch"=21011, "Smoothed Oval"=32500, "Smoothed Rounded Rectangle"=32505, "Sort 1D Array"=1120, "Sort Array of String"=23065, "Speed Of Light In Vacuum (m/sec)"=23518, "Spin Control (system)"=21900, "Split 1D Array"=1908, "Split Button"=21020, "Split Number"=1170, "Split Signals"=2351, "Spreadsheet String To Array"=1539, "Square"=23059, "Square Button"=3101, "Square LED (classic)"=3121, "Square LED (modern)"=21013, "Square Light"=3105, "Square Push Button"=3119, "Square Push Button (profile)"=3113, "Square Radio Button"=3107, "Square Root"=1060, "Stacked Sequence Structure"=2000, "Start TLS"=1731, "State"=2198, "State Diagram"=2051, "Static VI Reference"=2084, "Stop"=1350, "Stop Button"=21230, "String Constant"=2007, "String Control (classic)"=3200, "String Control (modern)"=21701, "String Control (system)"=21920, "String Indicator (classic)"=3201, "String Indicator (modern)"=21702, "String Length"=1502, "String Subset"=1503, "String To Byte Array"=1608, "String To IP"=1711, "String To Path"=1078, "String to Shared Variable"=1830, "Strip Path"=1420, "SubPanel"=21810, "SubPanel (Classic)"=21811, "SubPanel (NXG Style)"=21824, "SubPanel (System)"=21823, "Subtract"=1051, "Subtract (with error terminals)"=3916, "Swap Bytes"=1162, "Swap Values"=2401, "Swap Vector Element"=1912, "Swap Words"=1163, "Tab Constant"=23502, "Tab Control (classic)"=3330, "Tab Control (modern)"=3332, "Tab Control (NXG Style)"=32700, "Tab Control (system)"=3331, "Table (classic)"=21796, "Table (modern)"=21790, "Table (system)"=21797, "Tag Attribute Ring"=2063, "Tangent"=1202, "Tank (classic)"=3020, "Tank (modern)"=21006, "Target Structure"=2370, "TCP Close Connection"=1713, "TCP Create Listener"=1717, "TCP Flattened Read"=1718, "TCP Flattened Write"=1719, "TCP Flex Read"=1720, "TCP Flex Write"=1721, "TCP Network Connection Refnum"=3407, "TCP Open Connection"=1715, "TCP Read"=1716, "TCP Wait On Listener"=1712, "TCP Write"=1714, "TDMS Advanced Asynchronous Read (Data Ref)"=2151, "TDMS Advanced Asynchronous Write (Data Ref)"=2150, "TDMS Close"=24113, "TDMS Configure Asynchronous Reads (Data Ref)"=2153, "TDMS Configure Asynchronous Writes (Data Ref)"=2152, "TDMS Defragment"=24119, "TDMS Delete Data"=2159, "TDMS File"=3477, "TDMS Flush"=24117, "TDMS Get Asynchronous Read Status (Data Ref)"=2155, "TDMS Get Asynchronous Write Status (Data Ref)"=2154, "TDMS Get Properties"=24115, "TDMS In Memory Close"=2157, "TDMS In Memory Open"=2156, "TDMS In Memory Read Bytes"=2158, "TDMS List Contents"=24116, "TDMS Open"=24112, "TDMS Read"=24111, "TDMS Refnum To File ID"=24120, "TDMS Set Properties"=24114, "TDMS Write"=24110, "TDMS Write IP"=24118, "Temporary Directory"=1435, "TestSRQ"=1986, "TestSys"=1987, "Text & Pict Ring (classic)"=3016, "Text & Pict Ring (modern)"=21603, "Text Button"=21015, "Text Ring (block diagram constant)"=2008, "Text Ring (classic)"=3014, "Text Ring (modern)"=21601, "Text Ring (system)"=3060, "Text to UTF-8"=23066, "Thermometer (classic)"=3021, "Thermometer (modern)"=21007, "Threshold 1D Array"=1909, "Tick Count (ms)"=1300, "Time Stamp (block diagram constant)"=2068, "Time Stamp Control (classic)"=5555, "Time Stamp Control (modern)"=21913, "Time Stamp Control (system)"=21967, "Time Stamp Indicator (classic)"=5556, "Time Stamp Indicator (modern)"=21914, "Timed Loop"=5570, "Timed Sequence"=5573, "TLS Configuration"=3489, "TLS Connection?"=1740, "To Byte Integer"=1140, "To Double Precision Complex"=1152, "To Double Precision Float"=1147, "To Extended Precision Complex"=1154, "To Extended Precision Float"=1149, "To Fixed-Point"=5561, "To Long Integer"=1142, "To Lower Case"=1189, "To More Generic Class"=8017, "To More Specific Class"=8016, "To OLE Variant"=8002, "To Probe String"=2413, "To Quad Integer"=1155, "To Single Precision Complex"=1151, "To Single Precision Float"=1146, "To Time Stamp"=5560, "To Unsigned Byte Integer"=1143, "To Unsigned Long Integer"=1145, "To Unsigned Quad Integer"=1156, "To Unsigned Word Integer"=1144, "To Upper Case"=1188, "To Variant"=8201, "To Word Integer"=1141, "Traditional DAQ Channel (block diagram constant)"=2085, "Traditional DAQ Channel (classic)"=3320, "Traditional DAQ Channel (modern)"=21733, "Transpose 1D Array"=23068, "Transpose 2D Array"=1902, "Transpose Matrix"=8509, "Tree (classic)"=21819, "Tree (modern)"=21793, "Tree (system)"=21794, "Trigger"=1988, "TriggerList"=1989, "Two Button Dialog"=1341, "Type and Creator"=1434, "Type Cast"=1166, "Type Error"=2415, "Type Must Be Array"=2417, "Type Must Be Cluster"=2418, "Type Of"=2414, "Type Specialization Structure"=2373, "UDP Close"=1726, "UDP Multicast Open"=1727, "UDP Network Connection Refnum"=3418, "UDP Open"=1723, "UDP Read"=1724, "UDP Write"=1725, "Unbitpack from Array"=3136, "Unbundle"=2048, "Unbundle By Name"=2058, "Unflatten From JSON"=24202, "Unflatten From String"=1165, "Unflatten From XML"=8401, "Unleak Variant Value Reference"=2411, "Unpackage Matrix"=23000, "Unregister For Events"=2076, "Unregister Session"=2320, "Up Arrow"=3823, "Up Bow Valve (flat)"=3703, "Up Bow Valve (outline)"=3803, "Up Bow Valve (shaded)"=21763, "Up Rect Valve (flat)"=3702, "Up Rect Valve (outline)"=21762, "Up Rect Valve (shaded)"=3802, "Up Tee (flat)"=3812, "Up Tee (shaded)"=3712, "User Defined Refnum"=3428, "User Defined Refnum Tag (block diagram constant)"=3426, "User Defined Refnum Tag (classic)"=3429, "User Defined Refnum Tag (modern)"=21745, "User Defined Refnum Tag Flatten (classic)"=3454, "User Defined Refnum Tag Flatten (modern)"=21747, "User Defined Tag (block diagram constant)"=2114, "User Defined Tag (classic)"=3329, "User Defined Tag (modern)"=21749, "User Item"=3506, "UTF-8 to Text"=23067, "Variable Class Specifier Constant"=2106, "Variable Name Constant"=3478, "Variant"=3310, "Variant To Data"=8003, "Variant To Flattened String"=8203, "Vert Line"=3822, "Vert Pipe (flat)"=3816, "Vert Pipe (shaded)"=3716, "Vert Rocker"=21740, "Vertical Fill Slide (classic)"=3009, "Vertical Fill Slide (modern)"=21014, "Vertical Gradient Oval"=32501, "Vertical Gradient Rectangle"=32503, "Vertical Gradient Rounded Rectangle"=32506, "Vertical Graduated Bar"=21107, "Vertical Pointer Slide (classic)"=3007, "Vertical Pointer Slide (modern)"=21017, "Vertical Pointer Slide (system)"=21901, "Vertical Progress Bar (modern)"=21104, "Vertical Progress Bar (system)"=21909, "Vertical Scrollbar"=21111, "Vertical Slide (system)"=21903, "Vertical Slide Switch (classic)"=3115, "Vertical Slide Switch (modern)"=21741, "Vertical Smooth Box"=3634, "Vertical Splitter Bar"=21860, "Vertical Splitter Bar (Classic)"=21862, "Vertical Splitter Bar (NXG Style)"=21866, "Vertical Splitter Bar (System)"=21864, "Vertical Switch"=3109, "Vertical Toggle Switch (classic)"=3111, "Vertical Toggle Switch (modern)"=21005, "VI Library"=1425, "VI Refnum"=3422, "VI Server Reference"=2091, "VISA Assert Interrupt Signal"=2309, "VISA Assert Trigger"=1929, "VISA Assert Utility Signal"=2310, "VISA Clear"=1927, "VISA Close"=1922, "VISA Disable Event"=1940, "VISA Discard Events"=1941, "VISA Enable Event"=1942, "VISA Find Resource"=1923, "VISA Flush I/O Buffer"=2302, "VISA GPIB Command"=2315, "VISA GPIB Control ATN"=2316, "VISA GPIB Control REN"=2304, "VISA GPIB Pass Control"=2317, "VISA GPIB Send IFC"=2318, "VISA In 16"=1930, "VISA In 32"=1944, "VISA In 64"=2140, "VISA In 8"=1936, "VISA Lock"=1993, "VISA Map Address"=1932, "VISA Map Trigger"=2311, "VISA Memory Allocation"=1997, "VISA Memory Allocation Ex"=2146, "VISA Memory Free"=1998, "VISA Move"=2303, "VISA Move In 16"=1948, "VISA Move In 32"=1991, "VISA Move In 64"=2144, "VISA Move In 8"=1946, "VISA Move Out 16"=1949, "VISA Move Out 32"=1992, "VISA Move Out 64"=2145, "VISA Move Out 8"=1947, "VISA Open"=2308, "VISA Out 16"=1931, "VISA Out 32"=1945, "VISA Out 64"=2141, "VISA Out 8"=1937, "VISA Peek 16"=1934, "VISA Peek 32"=1995, "VISA Peek 64"=2142, "VISA Peek 8"=1938, "VISA Poke 16"=1935, "VISA Poke 32"=1996, "VISA Poke 64"=2143, "VISA Poke 8"=1939, "VISA Read"=1925, "VISA Read STB"=1928, "VISA Read To File"=2313, "VISA Refnum to Session"=2300, "VISA Resource Name"=3421, "VISA resource name (classic)"=3409, "VISA resource name (modern)"=21737, "VISA Set I/O Buffer Size"=2301, "VISA Status Description"=1924, "VISA Unlock"=1994, "VISA Unmap Address"=1933, "VISA Unmap Trigger"=2312, "VISA USB Control In"=2086, "VISA USB Control Out"=2087, "VISA VXI Cmd or Query"=2305, "VISA Wait on Event"=1943, "VISA Write"=1926, "VISA Write From File"=2314, "Volume Info"=1414, "Wait (ms)"=1302, "Wait For Activity"=1722, "Wait For Front Panel Activity"=1328, "Wait for GPIB RQS"=1952, "Wait on Notification"=9105, "Wait on Notification from Multiple"=9106, "Wait on Notification from Multiple with Notifier History"=9132, "Wait on Notification with Notifier History"=9131, "Wait on Occurrence"=1701, "Wait Until Next ms Multiple"=1327, "WaitSRQ"=1990, "Waveform Chart"=21010, "Waveform Chart (classic)"=3501, "Waveform Chart (modern)"=21717, "Waveform Graph (classic)"=3504, "Waveform Graph (modern)"=21703, "While Loop #1"=2003, "While Loop #2"=2352, "White Space?"=1125, "Write Datalog"=8079, "Write Device"=1431, "Write File"=1408, "Write Multiple Elements to Stream"=23804, "Write Single Element to Stream"=23798, "Write to Binary File"=8078, "Write to Text File"=8080, "Write Variable"=23782, "Write Variable with Timeout"=23789, "XY Graph (classic)"=3500, "XY Graph (modern)"=21716, "Y-th Root of X"=23062]
                            # "Create constant of the message's serialization cluster, to be wired to the cluster type of the subVI."
                            n52 = property class="VI"(reference=w235, error in=w224) -> (error out=w223:errorcluster, "Path"=w230:path)  [unwired: 1 out]
                            n53 = New VI Object(vi object class=w227, owner refnum=w234, style=w233, position/next to=T4 {"Horizontal"=0, "Vertical"=0} ("location"), 8:w223) -> (object refnum=w231:refnum<vi>, 0:w222:errorcluster)  [unwired: 3 in]
                            n54 = invoke class="ClustCnst" method="Replace"(reference=w231, error in=w222, "Path"=w230) -> (error out=w221:errorcluster, "Replace"=w228:refnum<vi>)  [unwired: 3 in, 4 out]
                            n55 = To More Specific Class(target class=w227, reference=w228, error in=w221) -> (specific class reference=w226:refnum<vi>, error out=w220:errorcluster)
                            n56 = property class="ClustCnst"(reference=w226, error in=w220) -> (error out=w219:errorcluster, "Terminal"=w225:refnum<vi>)  [unwired: 1 out]
                            n57 = call "Wire Two Terminals.vi"("error in (no error)"=w219, "Sink Terminal in"=w229, "Source Terminal"=w225) -> ("error out"=w218:errorcluster)  [unwired: 7 in, 1 out]
                          }
                        }
                      }
                      frame #2 {
                        # "Wire between the output of the subVI and the bundle node terminal."
                        n58 = call "Get Bundler Input Terminal By Name.vi"("error in (no error)"=w239, "Terminal name"=w248, "Bundler in"=w247) -> ("error out"=w238:errorcluster, "Found?"=w240:bool, "Terminal Refnum"=w244:refnum<vi>)  [unwired: 5 in, 1 out]
                        n59 = call "Get SubVI Terminal (by Name).vi"("error in (no error)"=w238, "Terminal name"="OutputCluster", "SubVI in"=w246) -> ("error out"=w237:errorcluster, "Found?"=w241:bool, "SubVI Term ref"=w243:refnum<vi>)  [unwired: 5 in, 1 out]
                        n60 = And(x=w241, y=w240) -> (x .and. y?=w242:bool)
                        n61 = case shown="True" w242 {
                          tunnel: w244 -> [_ w253]
                          tunnel: w243 -> [_ w252]
                          tunnel: w237 -> [w249 w251]
                          tunnel: [w249 w250] -> w236
                          frame False {
                          }
                          frame True {
                            n62 = call "Wire Two Terminals.vi"("error in (no error)"=w251, "Sink Terminal in"=w253, "Source Terminal"=w252) -> ("error out"=w250:errorcluster)  [unwired: 7 in, 1 out]
                          }
                        }
                      }
                    }
                  }
                }
              }
              frame Default {
                n63 = call "Get Bundler Input Terminal By Name.vi"("error in (no error)"=w260, "Terminal name"=w262, "Bundler in"=w255) -> ("error out"=w259:errorcluster, "Terminal Refnum"=w261:refnum<vi>)  [unwired: 5 in, 2 out]
                n64 = call "Get Unbundler Output Terminal By Name.vi"("error in (no error)"=w259, "Terminal name"=w262, "Unbundler in"=w254) -> ("error out"=w258:errorcluster, "Terminal Refnum"=w256:refnum<vi>)  [unwired: 5 in, 2 out]
                n65 = call "Wire Two Terminals.vi"("error in (no error)"=w258, "Sink Terminal in"=w256, "Source Terminal"=w261) -> ("error out"=w257:errorcluster)  [unwired: 7 in, 1 out]
              }
            }
          }
          frame True {
            # "Get the unbundle terminal whose name is <oneof container name>_selected_index.\nGet the bundle terminal whose name is <oneof container name> which is the class terminal."
            n66 = call "Get Bundler Input Terminal By Name.vi"("error in (no error)"=w273, "Terminal name"=w280, "Bundler in"=w298) -> ("error out"=w274:errorcluster, "Terminal Refnum"=w275:refnum<vi>)  [unwired: 5 in, 2 out]
            n67 = Concatenate Strings("Set" ("string"), w272, ".vi" ("string")) -> (w291:string)
            n68 = call "Get Case Structure (by Name).vi"("error in (no error)"=w274, "Case Structure name"=w280, "VI ref in"=w296) -> ("error out"=w286:errorcluster, "Found ?"=w294:bool, "CaseStructure out"=w287:refnum<vi>, "VI ref out"=w295:refnum<vi>)  [unwired: 5 in]
            n69 = case shown="False" w294 {
              tunnel: w297 -> [w373 w378]
              tunnel: w280 -> [w343 _]
              tunnel: w295 -> [w374 w376]
              tunnel: [w350 w379] -> w285
              tunnel: w287 -> [_ w379]
              tunnel: [w372 w378] -> w282
              tunnel: [w344 w377] -> w283
              tunnel: w286 -> [w369 w377]
              tunnel: [w366 w376] -> w269
              tunnel: w277 -> [w368 w375]
              tunnel: [w351 w375] -> w276
              tunnel: w275 -> [w353 _]
              frame False {
                n70 = call "Create Oneof Case Structure.vi"("error in (no error)"=w369, "Oneof Container Name"=w343, "VI in"=w374) -> ("error out"=w370:errorcluster, "CaseStructure out"=w371:refnum<vi>, "VI out"=w367:refnum<vi>)  [unwired: 6 in]
                n71 = Concatenate Strings(" \"" ("string"), w343, "\" " ("string")) -> (w342:string)
                n72 = call "Get Selected Index Terminal from Unbundler (by oneof name).vi"("error in (no error)"=w370, "Oneof Container Name"=w343, "Unbundler in"=w373) -> ("error out"=w357:errorcluster, "Terminal Refnum"=w360:refnum<vi>, "Unbundler out"=w372:refnum<vi>)  [unwired: 5 in, 1 out]
                n73 = call "Drop Protobuf To Field Converter SubVI.vi"("error in (no error)"=w357, "Oneof container name"=w343, "Owner VI in"=w367, "Library"=w368) -> ("error out"=w356:errorcluster, "SubVI out"=w365:refnum<vi>, "Owner VI out"=w366:refnum<vi>, "Library out"=w351:refnum<vi>)  [unwired: 4 in]
                n74 = call "Get SubVI Terminal (by Name).vi"("error in (no error)"=w356, "Terminal name"="protobuf index", "SubVI in"=w365) -> ("error out"=w355:errorcluster, "SubVI Term ref"=w359:refnum<vi>, "SubVI out"=w362:refnum<vi>)  [unwired: 5 in, 1 out]
                n75 = call "Wire Two Terminals.vi"("error in (no error)"=w355, "Sink Terminal in"=w359, "Source Terminal"=w360) -> ("error out"=w354:errorcluster)  [unwired: 7 in, 1 out]
                n76 = call "Get SubVI Terminal (by Name).vi"("error in (no error)"=w354, "Terminal name"="oneof field name", "SubVI in"=w362) -> ("error out"=w361:errorcluster, "SubVI Term ref"=w358:refnum<vi>)  [unwired: 5 in, 2 out]
                n77 = call "Connect Case Selector Terminal.vi"("error in (no error)"=w361, "Wire Source"=w358, "Case Structure in"=w371) -> ("error IO"=w348:errorcluster, "Case Structure out"=w350:refnum<vi>)  [unwired: 7 in]
                n78 = call "Drop Oneof Constant into Case Structure Default.vi"("error in (no error)"=w348, "Oneof Container Name"=w343, "CaseStructure in"=w350, "Library in"=w351) -> ("error out"=w349:errorcluster, "LVClass Constant Terminal out"=w352:refnum<vi>, "CaseStructure out"=w339:refnum<vi>)  [unwired: 4 in, 1 out]
                n79 = call "Wire Two Terminals.vi"("error in (no error)"=w349, "Sink Terminal in"=w353, "Source Terminal"=w352) -> ("error out"=w347:errorcluster, "Source Terminal out"=w346:refnum<vi>)  [unwired: 7 in]
                n80 = Close Reference(reference=w346, error in (no error)=w347) -> (error out=w345:errorcluster)
                n81 = call "Set Default Case By Frame Name.vi"("error in (no error)"=w345, "Frame Name"=w342, "CaseStructure in"=w339) -> ("error out"=w344:errorcluster)  [unwired: 7 in, 1 out]
              }
              frame True {
              }
            }
            n82 = call "Add Case Structure Frame (by Name).vi"("error in (no error)"=w283, "Frame name"=w272, "CaseStructure in"=w285) -> ("error out"=w264:errorcluster, "Case Frame"=w284:refnum<vi>, "CaseStructure out"=w271:refnum<vi>)  [unwired: 6 in]
            n83 = property class="VI"(reference=w269, error in=w264) -> (reference out=w267:refnum<vi>, error out=w263:errorcluster, "Path"=w266:path)
            n84 = call "Save VI at Path.vi"("error in (no error)"=w263, "Path"=w266, "VI in"=w267) -> ("error out"=w268:errorcluster, "VI out"=w265:refnum<vi>)  [unwired: 6 in, 1 out]
            n85 = call "Get Unbundler Output Terminal By Name.vi"("error in (no error)"=w268, "Terminal name"=w272, "Unbundler in"=w282) -> ("error out"=w270:errorcluster, "Terminal Refnum"=w281:refnum<vi>)  [unwired: 5 in, 2 out]
            n86 = call "Get VIRef from Library.vi"("error in (no error)"=w270, "Item Name"=w291, "Library"=w276) -> ("error out"=w279:errorcluster, "Found ?"=w292:bool, "VIref out"=w293:refnum<vi>, "Library"=w288:refnum<vi>)  [unwired: 5 in]
            n87 = case shown="True" w292 {
              tunnel: w293 -> [_ w338]
              tunnel: w284 -> [_ w336]
              tunnel: w281 -> [_ w332]
              tunnel: w279 -> [w299 w315]
              tunnel: [w299 w311] -> w278
              tunnel: w272 -> [_ w308]
              tunnel: w271 -> [_ w307]
              frame False {
              }
              frame True {
                # "Drop specific Setter VI"
                n88 = property class="VI"(reference=w338, error in=w315) -> (reference out=w312:refnum<vi>, error out=w316:errorcluster, "Path"=w337:path)
                n89 = Concatenate Strings(" \"" ("string"), w308, "\" " ("string")) -> (w302:string)
                n90 = call "Create SubVI.vi"("error in (no error)"=w316, "Path"=w337, "Diagram in"=w336) -> ("error out"=w318:errorcluster, "subVI refnum"=w335:refnum<vi>)  [unwired: 7 in]
                n91 = call "Get SubVI Terminal (by Name).vi"("error in (no error)"=w318, "Terminal name"="Set_Val", "SubVI in"=w335) -> ("error out"=w329:errorcluster, "SubVI Term ref"=w333:refnum<vi>, "SubVI out"=w331:refnum<vi>)  [unwired: 5 in, 1 out]
                n92 = call "Wire Two Terminals.vi"("error in (no error)"=w329, "Sink Terminal in"=w332, "Source Terminal"=w333) -> ("error out"=w330:errorcluster)  [unwired: 7 in, 1 out]
                n93 = call "Get SubVI Terminal (by Name).vi"("error in (no error)"=w330, "Terminal name"="OneOfTemplate out", "SubVI in"=w331) -> ("error out"=w304:errorcluster, "SubVI Term ref"=w306:refnum<vi>, "SubVI out"=w317:refnum<vi>)  [unwired: 5 in, 1 out]
                n94 = call "Find Frame Sink Terminal (Assuming only one sink).vi"("error in (no error)"=w304, "Frame Name"=w302, "CaseStructure in"=w307) -> ("error IO"=w303:errorcluster, "Terminal ref"=w305:refnum<vi>)  [unwired: 5 in, 2 out]
                n95 = call "Wire Two Terminals.vi"("error in (no error)"=w303, "Sink Terminal in"=w305, "Source Terminal"=w306) -> ("error out"=w324:errorcluster)  [unwired: 7 in, 1 out]
                n96 = call "Get SubVI Terminal (by Name).vi"("error in (no error)"=w324, "Terminal name"="OneOfTemplate in", "SubVI in"=w317) -> ("error out"=w323:errorcluster, "SubVI Term ref"=w326:refnum<vi>)  [unwired: 5 in, 2 out]
                n97 = invoke class="Term" method="Create Constant"(reference=w326, error in=w323, "Value"=variant) -> (reference out=w319:refnum<vi>, error out=w322:errorcluster, "Create Constant"=w321:refnum<vi>)  [unwired: 1 in, 1 out]
                n98 = property class="Const"(reference=w321, error in=w322) -> (reference out=w314:refnum<vi>, error out=w310:errorcluster, "Terminal"=w320:refnum<vi>)
                n99 = call "Wire Two Terminals.vi"("error in (no error)"=w310, "Sink Terminal in"=w319, "Source Terminal"=w320) -> ("error out"=w309:errorcluster)  [unwired: 7 in, 1 out]
                n100 = Close Reference(reference=w314, error in (no error)=w309) -> (error out=w313:errorcluster)
                n101 = Close Reference(reference=w312, error in (no error)=w313) -> (error out=w311:errorcluster)
              }
            }
          }
        }
      }
    }
  }
  "Library ref out" <- w1
  n102 = call "Cleanup VI BD.vi"("error in (no error)"=w15, "VI in"=w16) -> ("error out"=→"error IO":errorcluster, "VI out"=→"VI Refnum out":refnum<vi>)  [unwired: 8 in]
